vi "Read Stiffnesses in Summary.vi"(11 "StiffnessCalculator in":refnum<class "StiffnessCalculator.lvclass">) -> (2 "Stiffnesses in Summary":dbl[unit][](array[numeric]) min=-199630324.20594117 max=199630324.20594117 format="%.2f", 3 "StiffnessCalculator out":refnum<class "StiffnessCalculator.lvclass">)   [LabVIEW 2015, in "StiffnessCalculator.lvclass"]
uses:
  StiffnessCalculator.lvclass
  StiffnessCalculator.lvclass/StiffnessCalculator.ctl
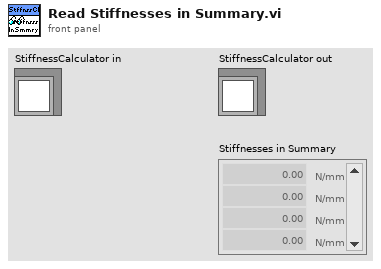
[diagram p1: front panel]
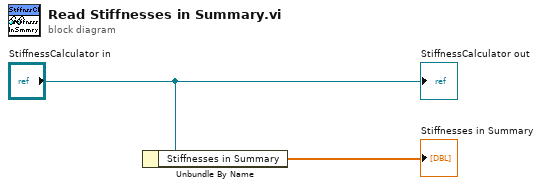
[diagram p0: block diagram]
diagram:
  n1 = Unbundle By Name("StiffnessCalculator in") -> ("Stiffnesses in Summary"=→"Stiffnesses in Summary":dbl[unit][])
  "StiffnessCalculator out" <- "StiffnessCalculator in"
